vi "Save Front Panel As Screenshot On Disk LV2012 NIVerified.vi"(7 "Image Type":enum16{"JPEG", "PNG", "BMP"}(ring), 8 "error in":errorcluster, 9 "Image Name":string="Front Panel", 10 "Image Folder":path, 11 "VI path":path) -> (0 "error out":errorcluster)   [LabVIEW 2017]
doc: "This VI demonstrates how to save the whole front panel of a VI as a screenshot on disk."
panel:
  # "Overview: Demonstrates how to save the whole front panel of a VI as a screenshot on disk.\nRequirements: LabVIEW Base Development System 2012 (or compatible)\nInstructions: \n1. Enter the path to a VI.\n2. Enter a folder for the image. Only select the folder.\n3. Enter the Image Name. You don't need to enter the file extension.\n4. Select the Image Type for the image.\n5. Run the VI.\n6. Open the image on disk."
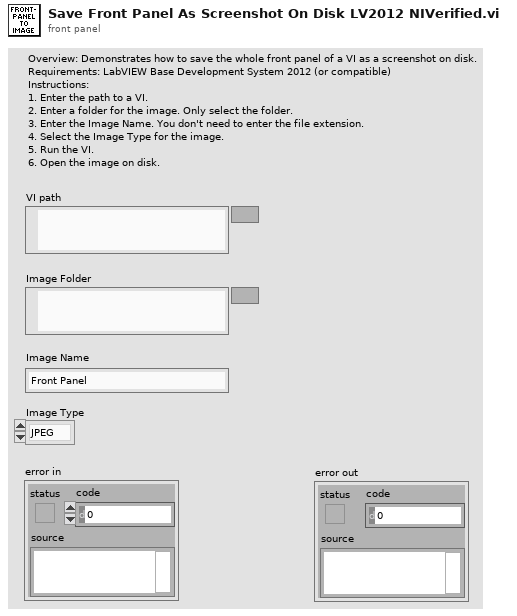
[diagram p1: front panel]
types:
  T1 = typedef "imagedata.ctl" = cluster{"image type":i32, "image depth":i32, "image":u8[], "mask":u8[], "colors":u32[], "Rectangle":cluster{"left":i16, "top":i16, "right":i16, "bottom":i16}}
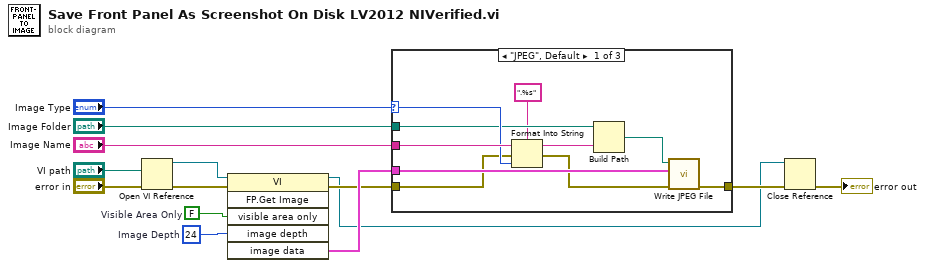
[diagram p0: block diagram]
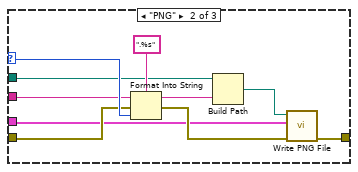
[diagram p2: hidden frame]
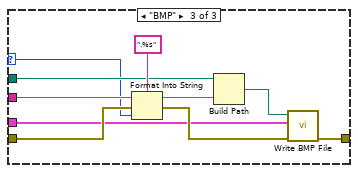
[diagram p3: hidden frame]
diagram:
  w13 = 24  # Image Depth
  w14 = FALSE  # Visible Area Only
  n1 = Open VI Reference(vi path="VI path", error in (no error)="error in") -> (vi reference=w12:refnum<vi>, error out=w11:errorcluster)  [unwired: 4 out]
  n2 = invoke class="VI" method="FP.Get Image"(reference=w12, error in=w11, "visible area only"=w14, "image depth"=w13) -> (reference out=w3:refnum<vi>, error out=w7:errorcluster, "image data"=w8:T1)  [unwired: 2 in, 3 out]
  n3 = case shown="\"JPEG\", Default" "Image Type" {
    selector: "Image Type" -> [w22 w32 w39]
    tunnel: w8 -> [w24 w27 w37]
    tunnel: w7 -> [w15 w29 w42]
    tunnel: [w17 w25 w36] -> w6
    tunnel: "Image Folder" -> [w21 w31 w40]
    tunnel: "Image Name" -> [w23 w30 w41]
    frame "JPEG", Default {
      n4 = Format Into String(format string=".%s", initial string=w23, error in=w15, w22) -> (resulting string=w20:string, error out=w16:errorcluster)
      n5 = Build Path(base path=w21, name or relative path=w20) -> (appended path=w18:path)
      n6 = call <vilib>:"Write JPEG File.vi"("error in (no error)"=w16, "image data"=w24, "path to JPEG file"=w18) -> ("error out"=w17:errorcluster)  [unwired: 8 out]
    }
    frame "PNG" {
      n7 = Format Into String(format string=".%s", initial string=w30, error in=w29, w32) -> (resulting string=w34:string, error out=w28:errorcluster)
      n8 = Build Path(base path=w31, name or relative path=w34) -> (appended path=w26:path)
      n9 = call <vilib>:"Write PNG File.vi"("error in (no error)"=w28, "image data"=w27, "path to PNG file"=w26) -> ("error out"=w25:errorcluster)  [unwired: 8 out]
    }
    frame "BMP" {
      n10 = Format Into String(format string=".%s", initial string=w41, error in=w42, w39) -> (resulting string=w44:string, error out=w38:errorcluster)
      n11 = Build Path(base path=w40, name or relative path=w44) -> (appended path=w35:path)
      n12 = call <vilib>:"Write BMP File.vi"("error in (no error)"=w38, "image data"=w37, "path to BMP file"=w35) -> ("error out"=w36:errorcluster)  [unwired: 8 out]
    }
  }
  n13 = Close Reference(reference=w3, error in (no error)=w6) -> (error out=→"error out":errorcluster)
